vi "Send Message and Wait for Reply.vi"(6 "Response Timeout(5000ms)":i32=5000, 7 "TcpRouter-Client in":refnum<class "TcpRouter-Client.lvclass">, 8 "error in (no error)":errorcluster, 9 "Target Module":string="Target", 10 "Arguments (\"\")":string, 11 "State":string="API State") -> (0 "error out":errorcluster, 2 "Response":string="DoA")   [LabVIEW 2020, in "CSM-TCP-Router.lvlib" / "TcpRouter-Client.lvclass"]
uses:
  TcpRouter-Client.lvclass
  _support/tcp-msg type.ctl
  f32241c3-0036-4787-bc41-e9c1f987f5e1.vi
  <userlib>/_NEVSTOP/Communicable State Machine(CSM)/AdvanceAPI/CSM - Revert Arguments-Safe String.vi
  <userlib>/_NEVSTOP/Communicable State Machine(CSM)/_Shared/Trim Single-line Text.vi
  <userlib>/_NEVSTOP/Communicable State Machine(CSM)/AdvanceAPI/CSM - Keywords.vi
  <userlib>/_NEVSTOP/Communicable State Machine(CSM)/_Polymophic/Build Synchronous Message with Arguments.vi
  CSM-TCP-Router.lvlib
  <userlib>/_NEVSTOP/Communicable State Machine(CSM)/Communicable State Machine.lvlib
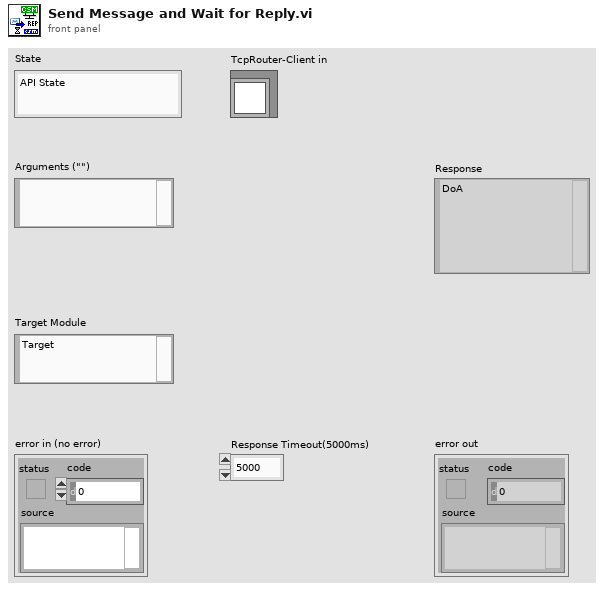
[diagram p1: front panel]
types:
  T1 = typedef "CSM-TCP-Router.lvlib/tcp-msg type.ctl" = enum8{"info", "error", "cmd", "cmd-resp", "resp", "async-resp", "status", "interrupt"}
  T2 = typedef "CSM-TCP-Router.lvlib/TcpRouter-Client.lvclass/Def-TCP-Router REQ-REP.ctl" = cluster{"REQ-REP":refnum<k5>}
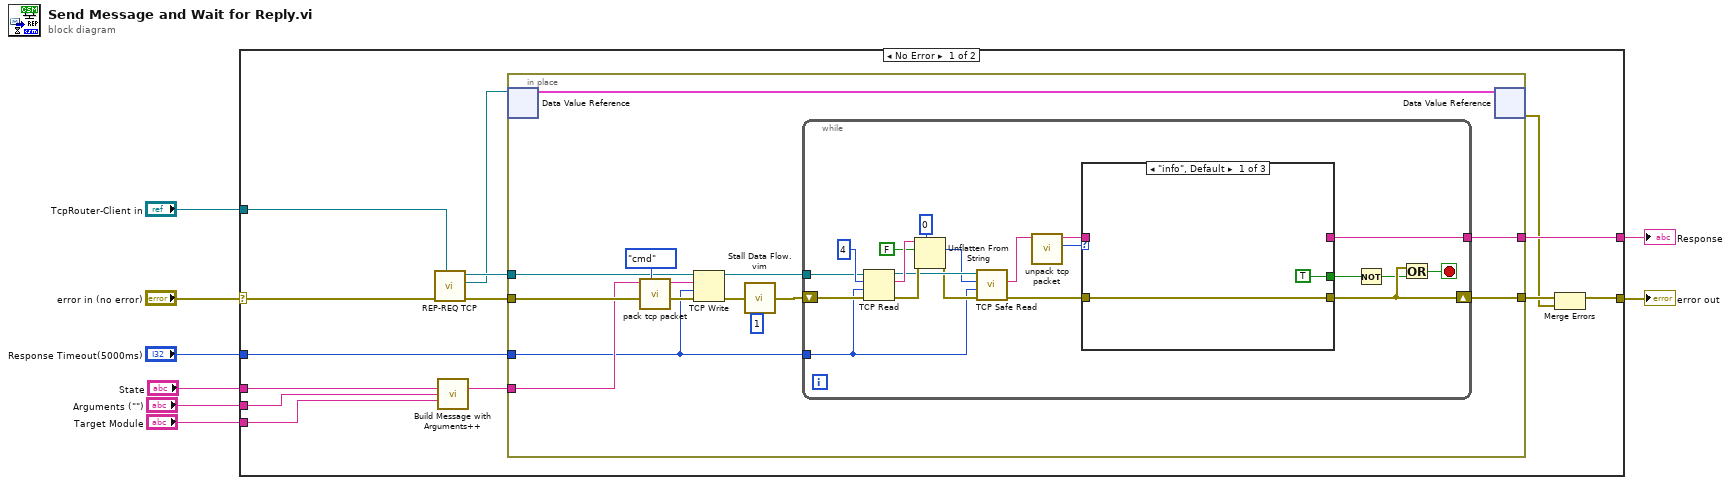
[diagram p0: block diagram]
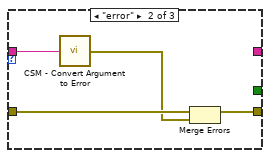
[diagram p2: hidden frame]
diagram:
  n1 = case shown="No Error" "error in (no error)" {
    selector: "error in (no error)" -> [w22 w64]
    tunnel: [w10 w64] -> w7
    tunnel: "TcpRouter-Client in" -> [w21 _]
    tunnel: "Response Timeout(5000ms)" -> [w12 _]
    tunnel: "State" -> [w18 _]
    tunnel: "Arguments (\"\")" -> [w17 _]
    tunnel: "Target Module" -> [w16 _]
    tunnel: [w13 _] -> w1
    frame No Error {
      n2 = call "REP-REQ TCP.vi"("TcpRouter-Client in"=w21, "error in (no error)"=w22) -> ("error out"=w20:errorcluster, "REQ-REP"=w11:refnum<data-value>, "connection ID"=w19:refnum<k5>)  [unwired: 7 in]
      n3 = call-poly <userlib>:"Build Message with Arguments++.vi"("State With Arguments"=w18, "Arguments (\"\")"=w17, "Target Module (\"\")"=w16) -> ("CSM Message String"=w15:string)  [unwired: 12 in]
      n4 = in-place {
        in-place-border: w20 -> [w33]
        in-place-border: w19 -> [w32]
        in-place-border: w15 -> [w31]
        in-place-border: [w26] -> w14
        in-place-border: [w25] -> w13
        in-place-border: w12 -> [w24]
        n5 = in-place-dvr #1(w11) -> (w23:T2)  [unwired: 1 out]
        n6 = call "pack tcp packet.vi"("tcp-message-type"=tcp-msg_type."cmd", "String"=w31) -> ("TCP Pack"=w35:string)  [unwired: 9 in]
        n7 = TCP Write(connection ID=w32, data in=w35, error in (no error)=w33, 9:w24) -> (connection ID out=w28:refnum<k5>, error out=w30:errorcluster)  [unwired: 1 out]
        n8 = call "Stall Data Flow.vim"("value in"=w30, "milliseconds to wait"=u32 1) -> ("value out"=w27:errorcluster)  [unwired: 1 out]
        n9 = while {
          tunnel: w28 -> [w46]
          tunnel: [w41] -> w25
          shift-right: [w40] -> w26
          shift-left: w27 -> [w45]
          tunnel: w24 -> [w39]
          stop <- w38 stop-if-true
          n10 = TCP Read(connection ID=w46, bytes to read=4, error in (no error)=w45, 9:w39) -> (connection ID out=w53:refnum<k5>, data out=w54:string, error out=w55:errorcluster)  [unwired: 1 in]
          n11 = Unflatten From String(type=0, binary string=w54, data includes array or string size? (T)=FALSE, error in (no error)=w55) -> (value=w51:i32, error out=w50:errorcluster)  [unwired: 2 out]
          n12 = call "TCP Safe Read.vi"("error in (no error)"=w50, "timeout ms (25000)"=w39, "bytes to read"=w51, "TCP Network Connection in"=w53) -> ("error out"=w43:errorcluster, "String"=w52:string)  [unwired: 5 in, 1 out]
          n13 = call "unpack tcp packet.vi"("TCP Pack"=w52) -> ("tcp-message-type"=w44:T1, "String"=w42:string)  [unwired: 9 in]
          n14 = case shown="\"info\", Default" w44 {
            tunnel: w43 -> [w57 w61 w63]
            tunnel: [w57 w59 w63] -> w40
            tunnel: w42 -> [_ w60 w62]
            tunnel: [_ _ w62] -> w41
            tunnel: [TRUE _ _] -> w37
            frame "info", Default {
            }
            frame "error" {
              n15 = call <userlib>:"CSM - Convert Argument to Error.vi"("Argument"=w60) -> ("Error"=w58:errorcluster)  [unwired: 4 in]
              n16 = Merge Errors(w61, w58) -> (w59:errorcluster)
            }
            frame "resp" {
            }
          }
          n17 = Not(x=w37) -> (.not. x?=w36:bool)
          n18 = Or(x=w40, y=w36) -> (x .or. y?=w38:bool)
        }
        n19 = in-place-dvr #1(w23) -> (w9:errorcluster)  [unwired: 1 out]
      }
      n20 = Merge Errors(w14, w9) -> (w10:errorcluster)
    }
    frame Error {
    }
  }
  "error out" <- w7
  "Response" <- w1
